vi "Extract OpenAI Response.vi"(0 "headers":string, 5 "body":string, 11 "error in":errorcluster) -> (4 "value":string, 15 "error out":errorcluster)   [LabVIEW 2020, in "llm_openai_chatmodels.lvclass"]
uses:
  llm_openai_chatmodels.lvclass
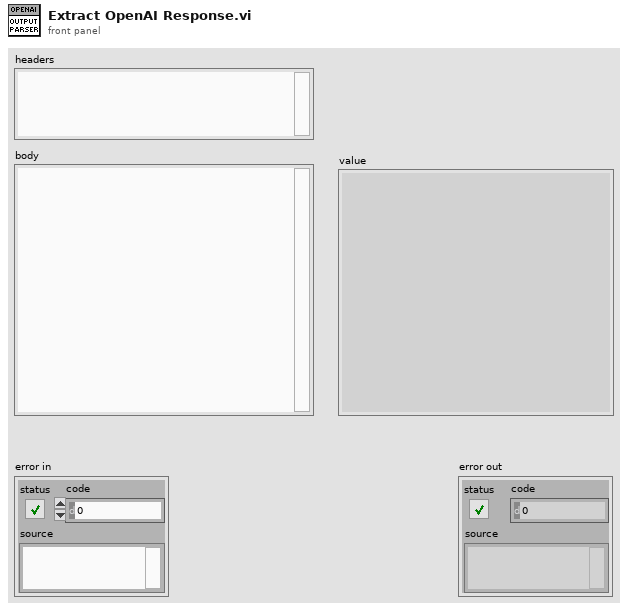
[diagram p1: front panel]
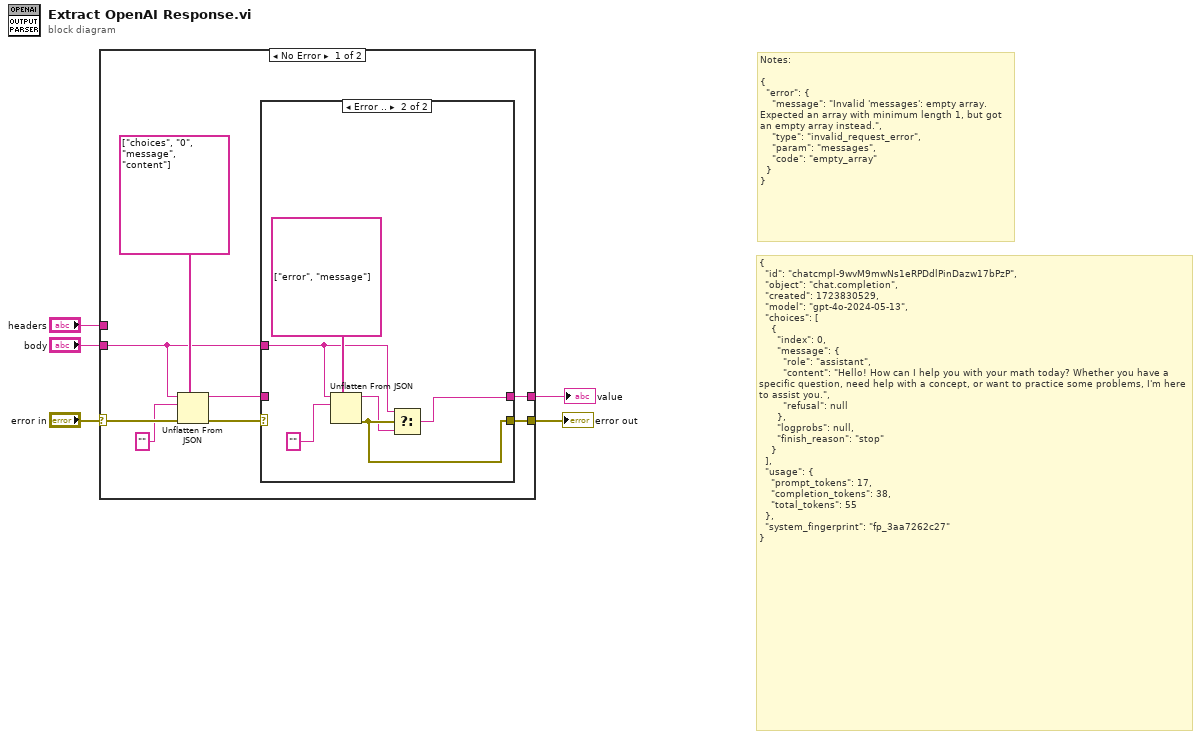
[diagram p0: block diagram]
diagram:
  # "{\n  \"id\": \"chatcmpl-9wvM9mwNs1eRPDdlPinDazw17bPzP\",\n  \"object\": \"chat.completion\",\n  \"created\": 1723830529,\n  \"model\": \"gpt-4o-2024-05-13\",\n  \"choices\": [\n    {\n      \"index\": 0,\n      \"message\": {\n        \"role\": \"assistant\",\n        \"content\": \"Hello! How can I help you with your math today? Whether you have a specific question, need help with a concept, or want to practice some problems, I'm here to assist you.\",\n        \"refusal\": null\n      },\n      \"logprobs\": null,\n      \"finish_reason\": \"stop\"\n    }\n  ],\n  \"usage\": {\n    \"prompt_tokens\": 17,\n    \"completion_tokens\": 38,\n    \"total_tokens\": 55\n  },\n  \"system_fingerprint\": \"fp_3aa7262c27\"\n}"
  # "Notes:\n\n{\n  \"error\": {\n    \"message\": \"Invalid 'messages': empty array. Expected an array with minimum length 1, but got an empty array instead.\",\n    \"type\": \"invalid_request_error\",\n    \"param\": \"messages\",\n    \"code\": \"empty_array\"\n  }\n}"
  n1 = case shown="No Error" "error in" {
    selector: "error in" -> [w13 w23]
    tunnel: [w9 w23] -> w4
    tunnel: "body" -> [w8 _]
    tunnel: "headers" -> [_ w22]
    tunnel: [w6 w22] -> w1
    frame No Error {
      n2 = Unflatten From JSON(path=string[] ["choices", "0", "message", "content"], JSON string=w8, type and defaults="", error in (no error)=w13) -> (value=w7:string, error out=w10:errorcluster)  [unwired: 3 in]
      n3 = case shown="Error .." w10 {
        selector: w10 -> [w15 _]
        tunnel: [w15 w18] -> w9
        tunnel: w8 -> [_ w16]
        tunnel: w7 -> [w14 _]
        tunnel: [w14 w19] -> w6
        frame No Error {
        }
        frame Error {
          n4 = Unflatten From JSON(path=string[] ["error", "message"], JSON string=w16, type and defaults="") -> (value=w17:string, error out=w18:errorcluster)  [unwired: 4 in]
          n5 = Select(t=w16, s=w18, f=w17) -> (s? t:f=w19:string)
        }
      }
    }
    frame Error {
    }
  }
  "error out" <- w4
  "value" <- w1
